vi "abort nanomessage.vi"(8 "error in":errorcluster) -> (0 "error out":errorcluster)   [LabVIEW 2013, in "lvnano.lvlib"]
doc: "NN_EXPORT void nn_term (void);"
uses:
  lvnano.lvlib
  lvnanomsg.dll
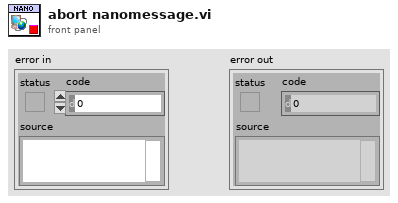
[diagram p1: front panel]
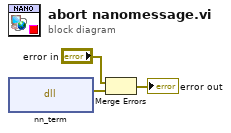
[diagram p0: block diagram]
diagram:
  n1 = dll-call lib="C:/Users/Daniel/Documents/nanomsg/lvnano/lvnanomsg.*" fn="nn_term"() -> (error out=w3:errorcluster)  [unwired: 4 in, 1 out]
  n2 = Merge Errors("error in", w3) -> (→"error out":errorcluster)
